vi "AccelnetVelOutScale.vi"(1 "Shaft vel (rpm)":dbl) -> (0 "Acelnet eCAT vel":i32)   [LabVIEW 2018]
uses:
  Clusters/SimulationConstants.ctl
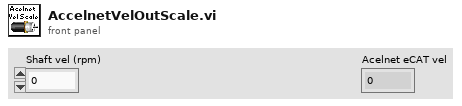
[diagram p1: front panel]
types:
  T1 = typedef "SimulationConstants.ctl" = cluster{"nGear":dbl, "rotorRadius":sgl, "numBlades":i32, "scaleFactor":dbl, "roscoInitMinSpeed_rad_s":dbl, "roscoInitMinTorqueFS_Nm":dbl, "beckhoff16bit":dbl, "beckhoff24BitExt":i32, "rotorTorqueScale_Nm_V":dbl, "rotorTorqueOfst_Nm":dbl, "rangeEL3104V":dbl, "nacelleAccELM3604V":dbl, "nacelleAccScaleX_m_s2_V":dbl, "nacelleAccOfstX_m_s2":dbl, "nacelleAccScaleY_m_s2_V":dbl, "nacelleAccOfstY_m_s2":dbl, "nacelleAccScaleZ_m_s2_V":dbl, "nacelleAccOfstZ_m_s2":dbl, "cyberGearRatio":dbl, "cyberLinesPerRev":dbl, "cyberRatedTorque":dbl, "towerTopForceScale":dbl, "towerTopTorqueScale":dbl, "plcSetpointScaling_norm2VFD":dbl, "towerBotScaleMy_Nm_V":dbl, "towerBotOfstMy_Nm":dbl, "towerTopScaleXaxis_N_V":dbl, "towerTopOfstXaxis_N":dbl, "towerTopScaleYaxis_N_V":dbl, "towerTopOfstYaxis_N":dbl, "pitchFlagOffset_deg":dbl, "anemWindSpeedScaleU_m_s_m_s":dbl, "anemWindSpeedOfstU_m_s":dbl, "anemWindSpeedScaleV_m_s_m_s":dbl, "anemWindSpeedOfstV_m_s":dbl, "anemWindSpeedScaleW_m_s_m_s":dbl, "anemWindSpeedOfstW_m_s":dbl, "anemWindSpeedScaleTSI1_m_s_V":dbl, "anemWindSpeedOfstTSI1_m_s":dbl}
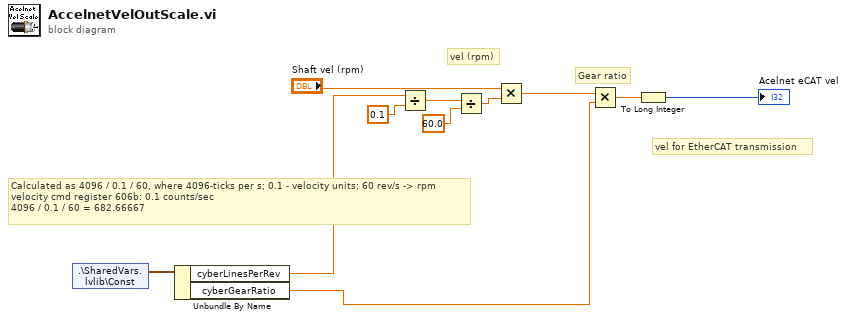
[diagram p0: block diagram]
diagram:
  # "vel for EtherCAT transmission"
  # "vel (rpm)"
  # "Calculated as 4096 / 0.1 / 60, where 4096-ticks per s; 0.1 - velocity units; 60 rev/s -> rpm\nvelocity cmd register 606b: 0.1 counts/sec\n4096 / 0.1 / 60 = 682.66667"
  # "Gear ratio"
  n1 = shared-variable ".\\SharedVars.lvlib\\Const"() -> (w8:T1)  [unwired: 1 in, 1 out]
  n2 = Unbundle By Name(w8) -> ("cyberLinesPerRev"=w1:dbl, "cyberGearRatio"=w2:dbl)
  n3 = Divide(x=w1, y=0.1) -> (x/y=w7:dbl)
  n4 = Divide(x=w7, y=60.0) -> (x/y=w3:dbl)
  n5 = Multiply(x="Shaft vel (rpm)", y=w3) -> (x*y=w4:dbl)
  n6 = Multiply(x=w4, y=w2) -> (x*y=w10:dbl)
  n7 = To Long Integer(number=w10) -> (32bit integer=→"Acelnet eCAT vel":i32)
